vi "ImagingGateSweep v1.2.vi"() -> ()   [LabVIEW 2021]
uses:
  <userlib>/Nanonis Prog Interface V5/Nanonis Prog Interface.lvlib
panel:
  in  "Time/Frame (s)":dbl
  in  "Tip move speed (m/s)":dbl=1e-09 format="%#_6p"
  in  "Home\nafter?":bool
  in  "milliseconds to wait":u32
  in  "Direction: \nUp\n\n\nDown":bool=TRUE
  in  "Serie name":string caption="Basename (empty= no change)"
  in  "Gate increment (V)":dbl
  in  "End gate (V)":dbl
  in  "Start gate (V)":dbl
  # "KPN: Correct Imaging vs. Gate voltage program, 8/9/22"
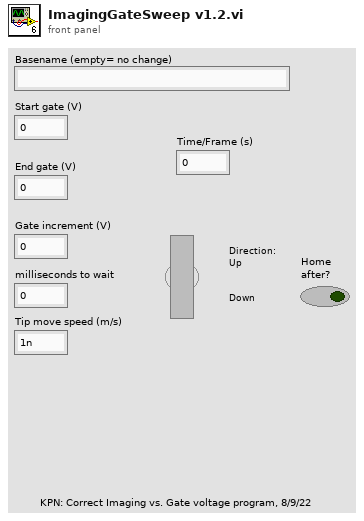
[diagram p1: front panel]
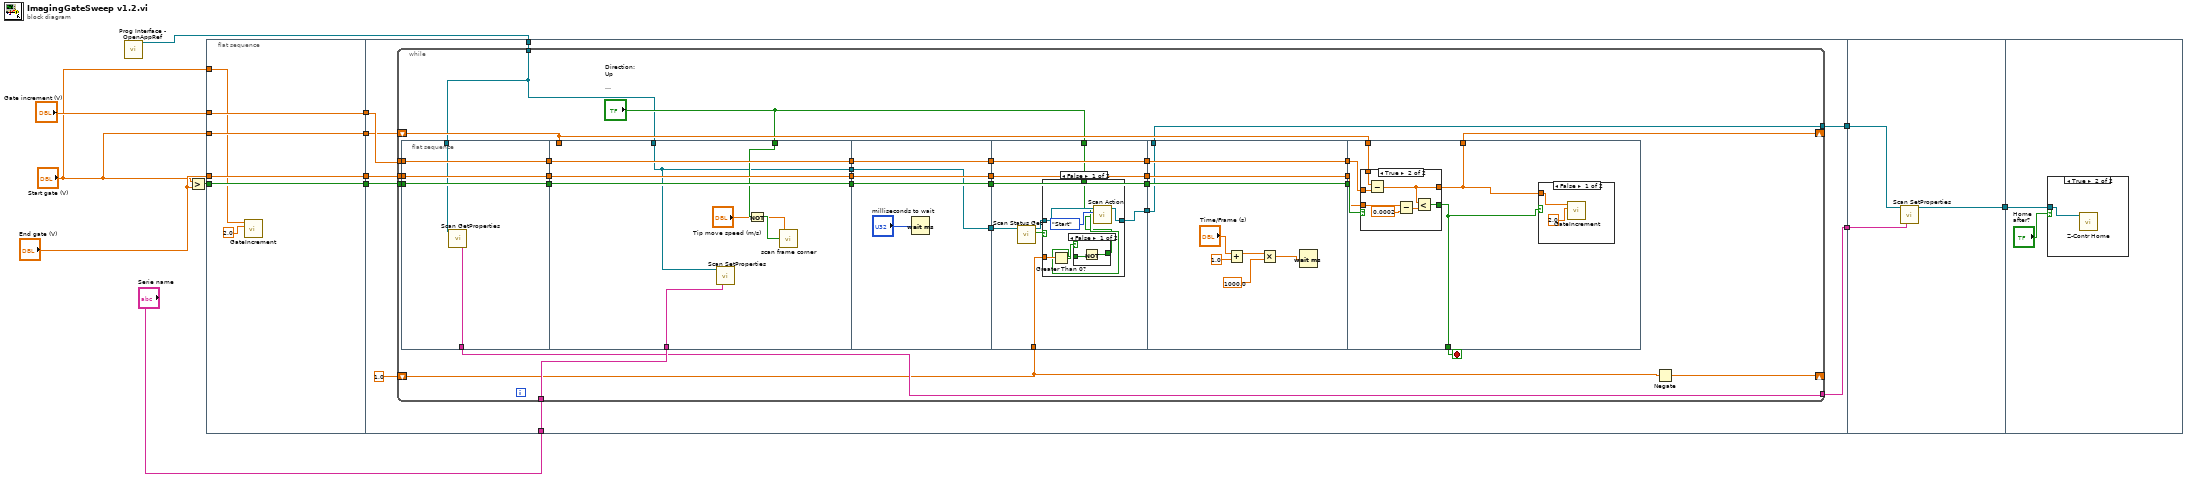
[diagram p0: block diagram]
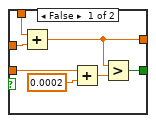
[diagram p5: hidden frame]
diagram:
  n1 = call <userlib>:"Prog Interface - OpenAppRef.vi"() -> ("Application reference"=w4:refnum<vi>)  [unwired: 6 in, 1 out]
  n2 = Greater?(x="Start gate (V)", y="End gate (V)") -> (0:w13:bool)
  n3 = flat-sequence {
    tunnel: "End gate (V)" -> [w16]
    tunnel: "Start gate (V)" -> [w17]
    tunnel: "Gate increment (V)" -> [w18]
    tunnel: w13 -> [w19]
    tunnel: [w19] -> w10
    tunnel: [w18] -> w9
    tunnel: [w17] -> w8
    tunnel: [w16] -> w7
    tunnel: "Start gate (V)" -> [w14]
    tunnel: w10 -> [w28]
    tunnel: w9 -> [w27]
    tunnel: w8 -> [w26]
    tunnel: w7 -> [w25]
    tunnel: w4 -> [w24]
    tunnel: "Serie name" -> [w23]
    tunnel: [w22] -> w2
    tunnel: [w21] -> w1
    tunnel: [w131] -> w3
    tunnel: w2 -> [w130]
    tunnel: w1 -> [w129]
    tunnel: w3 -> [w133]
    frame #0 {
      n4 = call "GateIncrement.vi"("Increment"=2.0, "Gate Voltage"=w14) -> ()  [unwired: 10 in]
    }
    frame #1 {
      n5 = while {
        tunnel: w28 -> [w59]
        tunnel: w27 -> [w58]
        shift-right: [w51] -> _
        shift-left: w26 -> [w52]
        tunnel: w25 -> [w57]
        tunnel: w24 -> [w31]
        tunnel: w23 -> [w53]
        tunnel: [w33] -> w22
        tunnel: [w32] -> w21
        shift-right: [w29] -> _
        shift-left: 1.0 -> [w30]
        stop <- w39 stop-if-true
        n6 = flat-sequence {
          tunnel: w59 -> [w62]
          tunnel: w58 -> [w63]
          tunnel: w57 -> [w64]
          tunnel: [w64] -> w36
          tunnel: [w63] -> w35
          tunnel: [w62] -> w34
          tunnel: [w61] -> w32
          tunnel: w31 -> [w60]
          tunnel: [w72] -> w50
          tunnel: [w71] -> w49
          tunnel: [w70] -> w48
          tunnel: "Direction: \nUp\n\n\nDown" -> [w69]
          tunnel: [w65] -> w37
          tunnel: w53 -> [w66]
          tunnel: w31 -> [w65]
          tunnel: w52 -> [_]
          tunnel: w36 -> [w70]
          tunnel: w35 -> [w71]
          tunnel: w34 -> [w72]
          tunnel: [w77] -> w46
          tunnel: [w76] -> w45
          tunnel: [w75] -> w44
          tunnel: w50 -> [w77]
          tunnel: w49 -> [w76]
          tunnel: w48 -> [w75]
          tunnel: [w73] -> w38
          tunnel: w37 -> [w73]
          tunnel: w46 -> [w86]
          tunnel: [w86] -> w43
          tunnel: w45 -> [w85]
          tunnel: [w85] -> w42
          tunnel: w44 -> [w84]
          tunnel: [w84] -> w41
          tunnel: [w83] -> w40
          tunnel: "Direction: \nUp\n\n\nDown" -> [w81]
          tunnel: w38 -> [w79]
          tunnel: w30 -> [w78]
          tunnel: [w106] -> w56
          tunnel: [w105] -> w55
          tunnel: [w104] -> w54
          tunnel: w40 -> [w98]
          tunnel: w41 -> [w104]
          tunnel: w42 -> [w105]
          tunnel: w43 -> [w106]
          tunnel: [w98] -> w33
          tunnel: w54 -> [w110]
          tunnel: w55 -> [w111]
          tunnel: w56 -> [w112]
          tunnel: [w109] -> w39
          tunnel: w52 -> [w108]
          tunnel: [w107] -> w51
          frame #0 {
            n7 = call <userlib>:"Scan GetProperties.vi"("Application ref in"=w60) -> ("Serie name"=w61:string)  [unwired: 7 in, 7 out]
          }
          frame #1 {
            n8 = call <userlib>:"Scan SetProperties.vi"("Application ref in"=w65, "Serie name"=w66) -> ()  [unwired: 12 in, 2 out]
            n9 = Not(x=w69) -> (.not. x?=w68:bool)
            n10 = call "scan frame corner.vi"("Speed (m/s)"="Tip move speed (m/s)", "Corner (T = top left, F = bottom left)"=w68) -> ()
          }
          frame #2 {
            n11 = Wait (ms)(milliseconds to wait="milliseconds to wait") -> ()  [unwired: 1 out]
          }
          frame #3 {
            n12 = call <userlib>:"Scan Status Get.vi"("Application ref in"=w79) -> ("Scanning?"=w82:bool, "Application ref out"=w80:refnum<vi>)  [unwired: 7 in, 1 out]
            n13 = case shown="False" w82 {
              tunnel: [w92 w97] -> w83
              tunnel: w81 -> [w88 _]
              tunnel: w80 -> [w91 w97]
              tunnel: w78 -> [w90 _]
              frame False {
                n14 = Greater Than 0?(x=w90) -> (x > 0?=w89:bool)
                n15 = case shown="False" w89 {
                  tunnel: w88 -> [w95 w96]
                  tunnel: [w94 w96] -> w87
                  frame False {
                    n16 = Not(x=w95) -> (.not. x?=w94:bool)
                  }
                  frame True {
                  }
                }
                n17 = call <userlib>:"Scan Action.vi"("Direction: up/down (T=up)"=w87, "Scan action (Start)"=enum16{"Start", "Stop", "Pause", "Resume"}."Start", "Application ref in"=w91) -> ("Application ref out"=w92:refnum<vi>)  [unwired: 6 in, 1 out]
              }
              frame True {
              }
            }
          }
          frame #4 {
            n18 = Add(x="Time/Frame (s)", y=1.0) -> (x+y=w101:dbl)
            n19 = Multiply(x=w101, y=1000.0) -> (x*y=w99:dbl)
            n20 = Wait (ms)(milliseconds to wait=w99) -> ()  [unwired: 1 out]
          }
          frame #5 {
            n21 = case shown="True" w112 {
              tunnel: w111 -> [w121 w128]
              tunnel: [w116 w126] -> w107
              tunnel: w110 -> [w120 w125]
              tunnel: [w118 w127] -> w109
              tunnel: w108 -> [w115 w122]
              frame False {
                n22 = Add(x=w115, y=w121) -> (x+y=w116:dbl)
                n23 = Add(x=w120, y=0.0002) -> (x+y=w117:dbl)
                n24 = Greater?(x=w116, y=w117) -> (0:w118:bool)
              }
              frame True {
                n25 = Subtract(x=w122, y=w128) -> (x-y=w126:dbl)
                n26 = Subtract(x=w125, y=0.0002) -> (x-y=w123:dbl)
                n27 = Less?(x=w126, y=w123) -> (x < y?=w127:bool)
              }
            }
            n28 = case shown="False" w109 {
              tunnel: w107 -> [w114 _]
              frame False {
                n29 = call "GateIncrement.vi"("Increment"=2.0, "Gate Voltage"=w114) -> ()  [unwired: 10 in]
              }
              frame True {
              }
            }
          }
        }
        n30 = Negate(x=w30) -> (-x=w29:dbl)
      }
    }
    frame #2 {
      n31 = call <userlib>:"Scan SetProperties.vi"("Application ref in"=w130, "Serie name"=w129) -> ("Application ref out"=w131:refnum<vi>)  [unwired: 12 in, 1 out]
    }
    frame #3 {
      n32 = case shown="True" "Home\nafter?" {
        tunnel: w133 -> [_ w134]
        frame False {
        }
        frame True {
          n33 = call <userlib>:"Z-Contr Home.vi"("Application ref in"=w134) -> ()  [unwired: 9 in, 2 out]
        }
      }
    }
  }
